vi "FPGA Write Inputs.vi"(8 "error in (no error)":errorcluster, 11 "Acquisition Loop Data in":T1) -> (0 "error out":errorcluster)   [LabVIEW 2018]
uses:
  <vilib>/rvi/interface/nirviReadWriteControl/nirviReadWriteControl.xnode
  FPGA/FPGA VI Reference.ctl
  NiFpgaLv.dll
  <vilib>/Utility/error.llb/Error Cluster From Error Code.vi
  <vilib>/rvi/interface/Simulation/niFpgaSimulationCallBeginRW.vi
  <vilib>/rvi/errors/niLvFpgaAdjustHostInterfaceError.vi
  Private Controls/Acquisition Loop Data.ctl
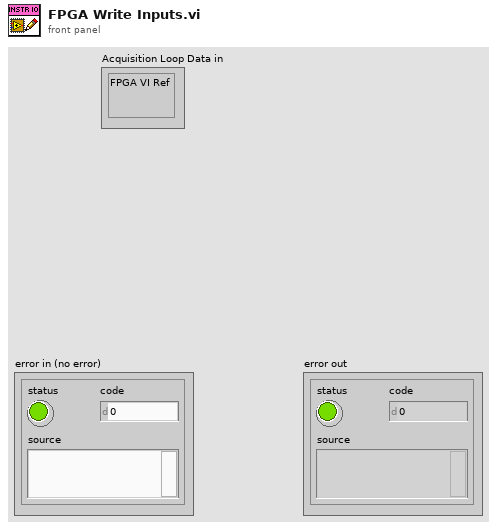
[diagram p1: front panel]
types:
  T1 = typedef "RT - Instrument IO.lvlib/Acquisition Loop Data.ctl" = cluster{"FPGA VI Ref":T2}
  T2 = typedef "FPGA VI Reference.ctl" = refnum<k20>
  T3 = typedef "RT - Instrument IO.lvlib/FPGA Write Queue Data.ctl" = cluster{"Input Data? (T)":bool, "Input Data":T4, "Overspeed Thresholds (RPM)":sgl[]}
  T4 = typedef "DAQ Input Data.ctl" = cluster{"00-04-9265 Vals":sgl[]}
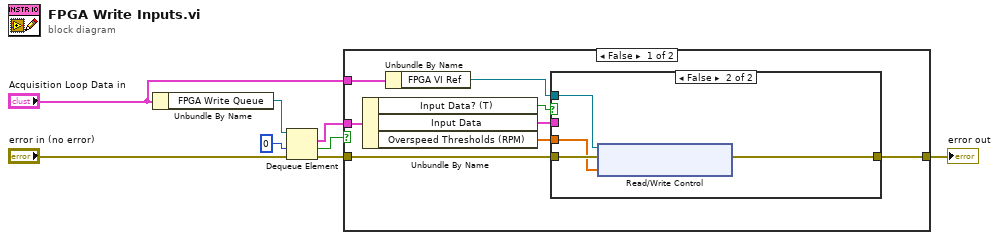
[diagram p0: block diagram]
diagram:
  n1 = Unbundle By Name("Acquisition Loop Data in") -> ("FPGA Write Queue"=w3:refnum<queue>)
  n2 = Dequeue Element(queue=w3, timeout in ms (-1)=0, error in (no error)="error in (no error)") -> (element=w6:T3, timed out?=w5:bool, error out=w1:errorcluster)  [unwired: 1 out]
  n3 = case shown="False" w5 {
    tunnel: "Acquisition Loop Data in" -> [w16 _]
    tunnel: w1 -> [w13 w21]
    tunnel: [w14 w21] -> w8
    tunnel: w6 -> [w12 _]
    frame False {
      n4 = Unbundle By Name(w12) -> ("Input Data? (T)"=w11:bool, "Input Data"=w10:T4, "Overspeed Thresholds (RPM)"=w9:sgl[])
      n5 = Unbundle By Name(w16) -> ("FPGA VI Ref"=w15:T2)
      n6 = case shown="False" w11 {
        tunnel: w15 -> [_ w20]
        tunnel: [_ w19] -> w14
        tunnel: w13 -> [_ w18]
        tunnel: w10 -> [_ _]
        tunnel: w9 -> [_ w17]
        frame True {
        }
        frame False {
          n7 = xnode "Read/Write Control"("FPGA VI Reference In"=w20, "error in"=w18, "Overspeed Thresholds"=w17) -> ("error out"=w19:errorcluster)  [unwired: 1 out]
        }
      }
    }
    frame True {
      # "Nothing in Queue, so don't do anything"
    }
  }
  "error out" <- w8
